vi "Read CSV File.vi"(8 "error in":errorcluster, 11 "File Path":path) -> (0 "error out":errorcluster, 3 "Data Out":dbl[][](array[numeric]) format="%0.2f")   [LabVIEW 2021]
doc: "Reads data from a .csv file."
uses:
  <vilib>/Utility/file.llb/Read Delimited Spreadsheet (DBL).vi
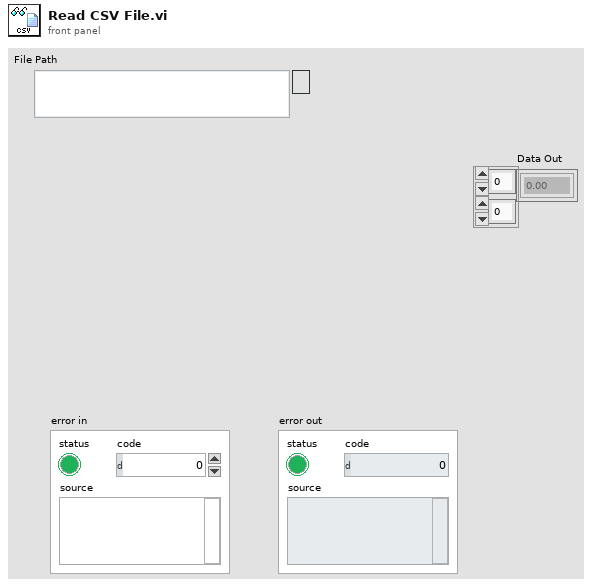
[diagram p1: front panel]
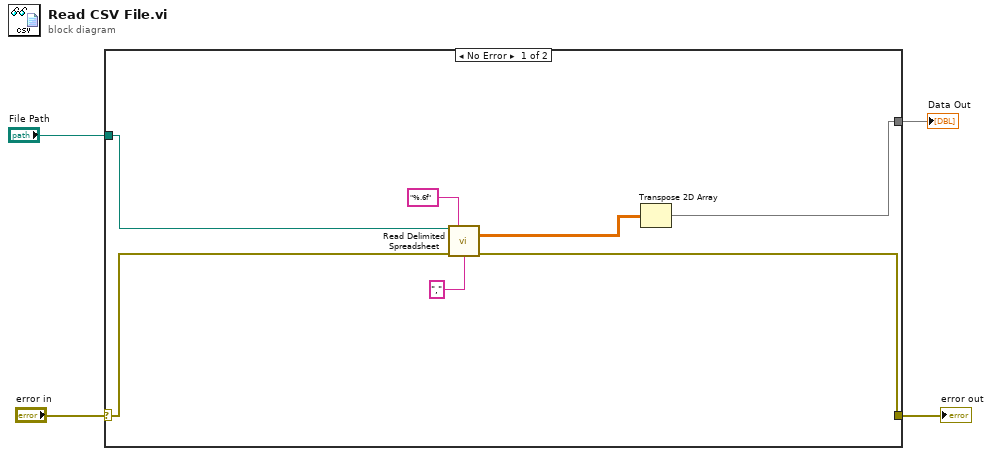
[diagram p0: block diagram]
diagram:
  n1 = case shown="No Error" "error in" {
    selector: "error in" -> [w11 w12]
    tunnel: "File Path" -> [w10 _]
    tunnel: [w8 w12] -> w2
    tunnel: [w5 _] -> w1
    frame No Error {
      n2 = call-poly <vilib>:"Read Delimited Spreadsheet.vi"("file path (dialog if empty)"=w10, "format (%.3f)"="%.6f", "error in (no error)"=w11, "delimiter (\\t)"="," ("delimiter (\\t)")) -> ("all rows"=w6:dbl[][], "error out"=w8:errorcluster)  [unwired: 6 in, 4 out]
      n3 = Transpose 2D Array(2D array=w6) -> (transposed array=w5:dbl[][])
    }
    frame Error {
    }
  }
  "error out" <- w2
  "Data Out" <- w1
